vi "rad_Configure Targets Settings Dialog.vi"(11 "Targets Settings":T1) -> (1 "Cancelled":bool, 3 "Targets Settings":T1)   [LabVIEW 2013]
uses:
  TypeDefs/rad_Targets Settings.ctl
  Util/FP Control/FP Control Functions.ctl
panel:
  in  "Reduce Discovery\nTimeout":bool
  in  "Other":bool
  in  "User Targets Only":bool
  in  "PXI":bool
  in  "FP":bool
  in  "cRIO":bool
  in  "Cancel":bool
  in  "OK":bool
  # "Targets to Display"
  # "Target Types"
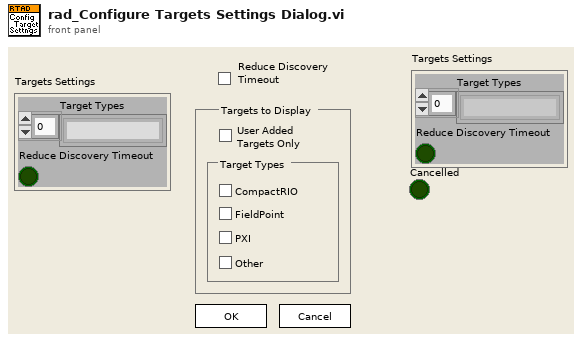
[diagram p1: front panel]
types:
  T1 = typedef "rad_Targets Settings.ctl" = cluster{"Target Types":string[], "Reduce Discovery Timeout":bool}
  T2 = typedef "FP Control Functions.ctl" = enum16{"Open", "Close", "Bring To Front", "Center"}
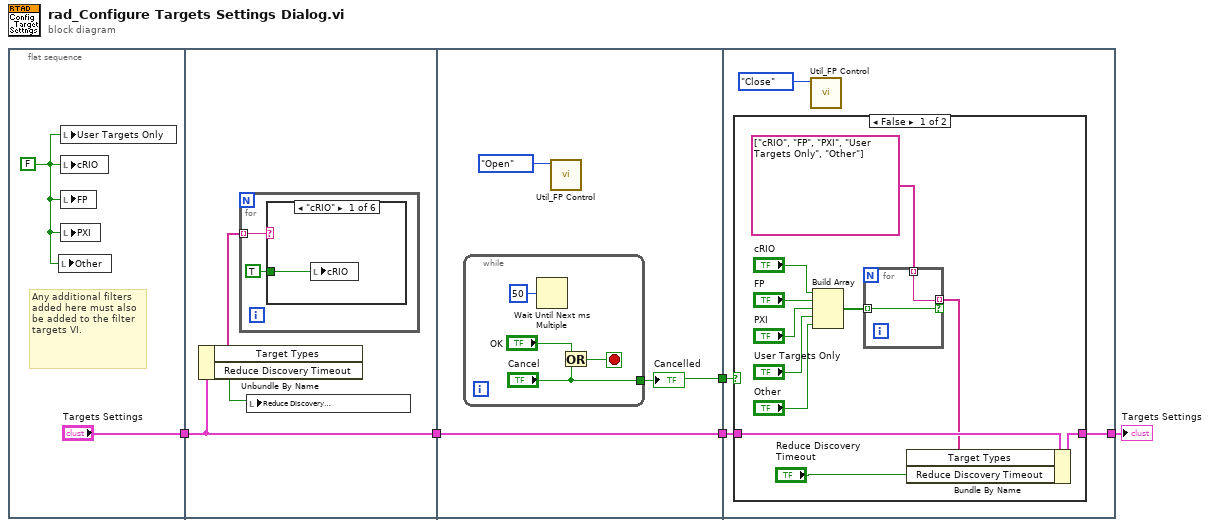
[diagram p0: block diagram]
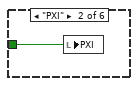
[diagram p2: hidden frame]
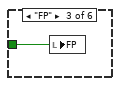
[diagram p3: hidden frame]
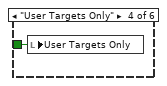
[diagram p4: hidden frame]
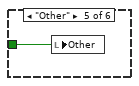
[diagram p5: hidden frame]
diagram:
  n1 = flat-sequence {
    tunnel: ["Targets Settings"] -> w1
    tunnel: [w10] -> w2
    tunnel: w1 -> [w10]
    tunnel: [w20] -> w5
    tunnel: [w19] -> w4
    tunnel: w2 -> [w19]
    tunnel: w5 -> [w28]
    tunnel: w4 -> [w27]
    tunnel: [w26] -> w3
    frame #0 {
      w6 = FALSE
      # "Any additional filters added here must also be added to the filter targets VI."
      n2 = local write "Other"(w6) -> ()
      n3 = local write "User Targets Only"(w6) -> ()
      n4 = local write "cRIO"(w6) -> ()
      n5 = local write "FP"(w6) -> ()
      n6 = local write "PXI"(w6) -> ()
    }
    frame #1 {
      n7 = Unbundle By Name(w10) -> ("Target Types"=w9:string[], "Reduce Discovery Timeout"=w8:bool)
      n8 = for {
        tunnel: w9 -> [w12] mode=indexing
        n9 = case shown="\"cRIO\"" w12 {
          tunnel: TRUE -> [w13 w14 w15 w16 w17 _]
          frame "cRIO" {
            n10 = local write "cRIO"(w13) -> ()
          }
          frame "PXI" {
            n11 = local write "PXI"(w14) -> ()
          }
          frame "FP" {
            n12 = local write "FP"(w15) -> ()
          }
          frame "User Targets Only" {
            n13 = local write "User Targets Only"(w16) -> ()
          }
          frame "Other" {
            n14 = local write "Other"(w17) -> ()
          }
          frame Default {
          }
        }
      }
      n15 = local write "Reduce Discovery\nTimeout"(w8) -> ()
    }
    frame #2 {
      n16 = while {
        tunnel: ["Cancel"] -> w20
        stop <- w22 stop-if-true
        n17 = Wait Until Next ms Multiple(millisecond multiple=u32 50) -> ()  [unwired: 1 out]
        n18 = Or(x="OK", y="Cancel") -> (x .or. y?=w22:bool)
      }
      "Cancelled" <- w20
      n19 = call "Util_FP Control.vi"("Function"=FP_Control_Functions."Open") -> ()  [unwired: 1 in, 10 out]
    }
    frame #3 {
      n20 = case shown="False" w28 {
        tunnel: w27 -> [w34 w42]
        tunnel: [w33 w42] -> w26
        frame False {
          n21 = Build Array("cRIO", "FP", "PXI", "User Targets Only", "Other") -> (w36:bool[])
          n22 = for {
            tunnel: w36 -> [w40] mode=indexing
            tunnel: string[] ["cRIO", "FP", "PXI", "User Targets Only", "Other"] -> [w41] mode=indexing
            tunnel: [w41] -> w29 mode=indexing if=w40
          }
          n23 = Bundle By Name(cluster=w34, "Target Types"=w29, "Reduce Discovery Timeout"="Reduce Discovery\nTimeout") -> (w33:T1)
        }
        frame True {
        }
      }
      n24 = call "Util_FP Control.vi"("Function"=FP_Control_Functions."Close") -> ()  [unwired: 1 in, 10 out]
    }
  }
  "Targets Settings" <- w3
